vi "GetParam.vi"(8 "error in (no error)":errorcluster caption="entrée d'erreur (pas d'erreur)", 11 "Average_Precision_Score.lvclass":refnum<class "Average_Precision_Score.lvclass">) -> (0 "error out":errorcluster caption="sortie d'erreur", 2 "average_precision_score":T1={"average"="macro", "pos_label"={"dtype_pos_label"="int", "pos_label"="1"}, "sample_weight"=[]}, 3 "Average_Precision_Score.lvclass":refnum<class "Average_Precision_Score.lvclass">)   [LabVIEW 2020, in "Average_Precision_Score.lvclass"]
doc: "Get Parameters"
uses:
  Average_Precision_Score.lvclass
  Average_Precision_Score.lvclass/Average_Precision_Score.ctl
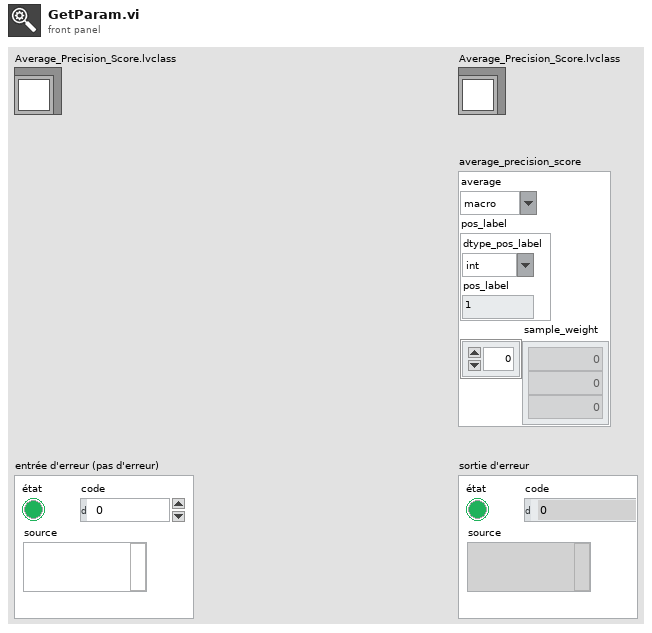
[diagram p1: front panel]
types:
  T1 = cluster{"average":string, "pos_label":cluster{"dtype_pos_label":string, "pos_label":string}, "sample_weight":dbl[]}
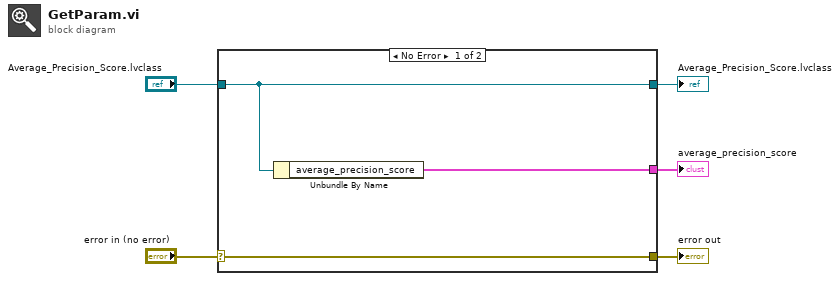
[diagram p0: block diagram]
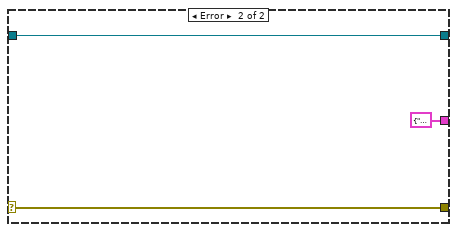
[diagram p2: hidden frame]
diagram:
  n1 = case shown="No Error" "error in (no error)" {
    selector: "error in (no error)" -> [w8 w10]
    tunnel: [w8 w10] -> w4
    tunnel: [w7 w11] -> w2
    tunnel: "Average_Precision_Score.lvclass" -> [w7 w11]
    tunnel: [w6 T1 {"average"="", "pos_label"={"dtype_pos_label"="", "pos_label"=""}, "sample_weight"=[]} ("average_precision_score")] -> w1
    frame No Error {
      n2 = Unbundle By Name(w7) -> ("average_precision_score"=w6:T1)
    }
    frame Error {
    }
  }
  "error out" <- w4
  "Average_Precision_Score.lvclass" <- w2
  "average_precision_score" <- w1
